vi "Create Data File.vi"(8 "Error In":errorcluster) -> (0 "Error Out":errorcluster, 3 "File Refnum":refnum<file>)   [LabVIEW 2018]
doc: "This VI performs a series of tasks to create a file for logging data:\n\n1) Check to see if a folder called 'Logged Data' exsists in the same directory as the application\n2) If the folder does not exsist, create it\n3) Create a file name of the format 'Acquired Data <Date> <Time>.txt'\n4) Replace or Create the file"
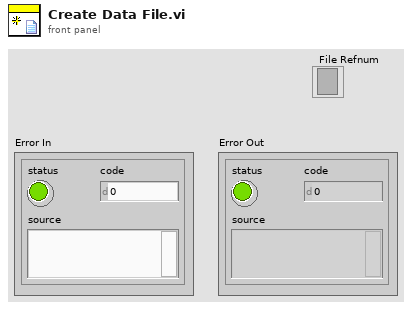
[diagram p1: front panel]
types:
  T1 = enum16{"open", "replace", "create", "open or create", "replace or create", "replace or create with confirmation"}
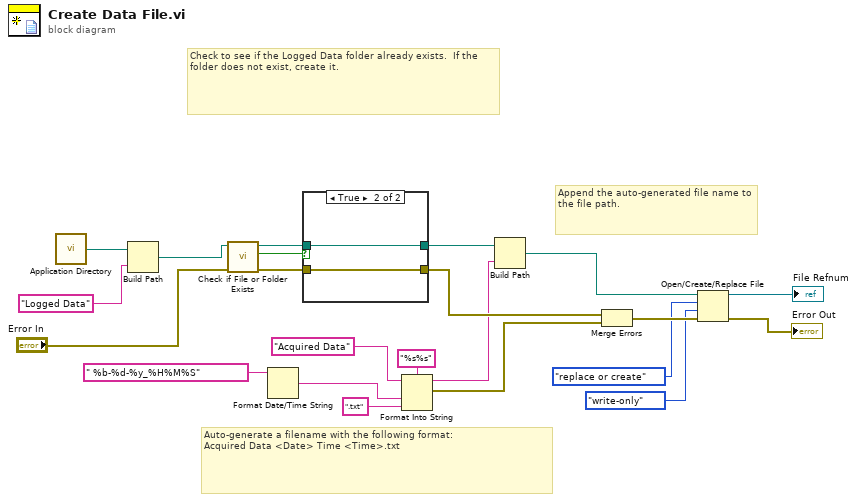
[diagram p0: block diagram]
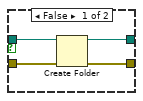
[diagram p2: hidden frame]
diagram:
  # "Append the auto-generated file name to the file path."
  # "Check to see if the Logged Data folder already exists.  If the folder does not exist, create it."
  # "Auto-generate a filename with the following format:\nAcquired Data <Date> Time <Time>.txt"
  n1 = call <vilib>:"Application Directory.vi"() -> ("Application Directory"=w13:path)
  n2 = Build Path(base path=w13, name or relative path="Logged Data" ("prompt (Create Folder)")) -> (appended path=w3:path)
  n3 = call <vilib>:"Check if File or Folder Exists.vi"("error in (no error)"="Error In", "path"=w3) -> ("error out"=w4:errorcluster, "file or folder exists?"=w1:bool, "dup path"=w2:path)  [unwired: 7 in]
  n4 = Format Date/Time String(time format string (%c)=" %b-%d-%y_%H%M%S") -> (date/time string=w9:string)  [unwired: 2 in]
  n5 = case shown="True" w1 {
    tunnel: [w23 w28] -> w16
    tunnel: [w26 w27] -> w15
    tunnel: w4 -> [w25 w27]
    tunnel: w2 -> [w24 w28]
    frame False {
      n6 = Create Folder(path (use dialog)=w24, error in=w25) -> (created path=w23:path, error out=w26:errorcluster)  [unwired: 1 in, 1 out]
    }
    frame True {
    }
  }
  n7 = Format Into String(format string="%s%s", initial string="Acquired Data" ("string"), w9, ".txt" ("string")) -> (resulting string=w6:string, error out=w7:errorcluster)  [unwired: 1 in]
  n8 = Build Path(base path=w16, name or relative path=w6) -> (appended path=w22:path)
  n9 = Merge Errors(w15, w7) -> (w21:errorcluster)
  n10 = Open/Create/Replace File(file path (use dialog)=w22, error in=w21, operation (0:open)=T1."replace or create", access (0:read/write)=enum16{"read/write", "read-only", "write-only"}."write-only") -> (refnum out=→"File Refnum":refnum<file>, error out=→"Error Out":errorcluster)  [unwired: 2 in, 1 out]
